vi "synchronize capture with burst.vi"(8 "error in (no error)":errorcluster, 10 "Image Array":T1[](array[typedef]), 11 "Refnum in":T2) -> (0 "error out":errorcluster, 3 "Refnum out":T2)   [LabVIEW 2020]
uses:
  <vilib>/userdefined/High Color/IMAQdx.ctl
  <vilib>/vision/Image Controls.llb/IMAQ Image.ctl
  <vilib>/vision/driver/IMAQdx.llb/IMAQdx Acquisition Mode.ctl
  <vilib>/vision/driver/IMAQdx.llb/IMAQdx Buffer Number Mode.ctl
  <vilib>/vision/driver/NI_Vision_Acquisition_Software.lvlib
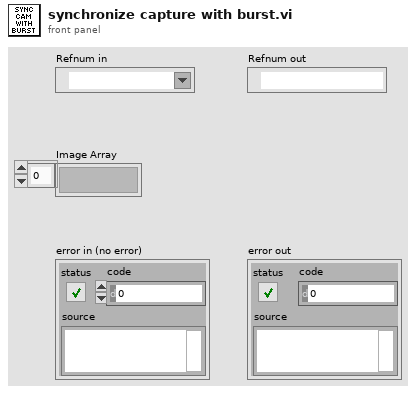
[diagram p1: front panel]
types:
  T1 = typedef "IMAQ Image.ctl" = refnum<image>
  T2 = typedef "IMAQdx.ctl" = refnum<k21>
  T3 = typedef "NI_Vision_Acquisition_Software.lvlib/IMAQdx Acquisition Mode.ctl" = enum32{"One Shot", "Continuous"}
  T4 = typedef "NI_Vision_Acquisition_Software.lvlib/IMAQdx Buffer Number Mode.ctl" = enum32{"Next", "Last", "Buffer Number", "Every", "Last New"}
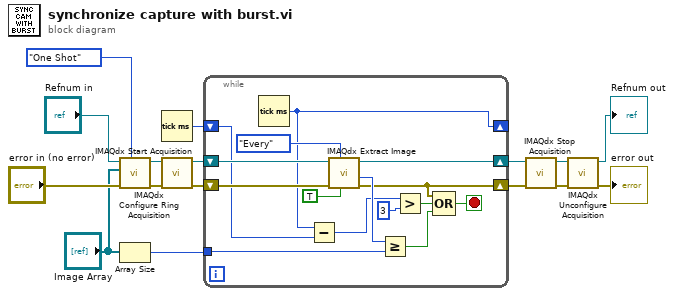
[diagram p0: block diagram]
diagram:
  n1 = call <vilib>:"IMAQdx Configure Ring Acquisition.vi"("Mode"=IMAQdx_Acquisition_Mode."One Shot" ("Continuous?"), "error in"="error in (no error)", "Images"="Image Array", "Session In"="Refnum in") -> ("error out"=w11:errorcluster, "Session Out"=w10:T2)  [unwired: 5 in, 1 out]
  n2 = Array Size(array="Image Array") -> (size(s)=w8:i32)
  n3 = Tick Count (ms)() -> (millisecond timer value=w9:u32)
  n4 = call <vilib>:"IMAQdx Start Acquisition.vi"("error in"=w11, "Session In"=w10) -> ("error out"=w14:errorcluster, "Session Out"=w15:T2)  [unwired: 8 out]
  n5 = while {
    shift-right: [w31] -> w4
    shift-left: w15 -> [w30]
    shift-right: [w17] -> w2
    shift-left: w14 -> [w29]
    shift-right: [w24] -> _
    shift-left: w9 -> [w23]
    tunnel: w8 -> [w25]
    stop <- w18 stop-if-true
    n6 = Tick Count (ms)() -> (millisecond timer value=w24:u32)
    n7 = Subtract(x=w24, y=w23) -> (x-y=w22:u32)
    n8 = call <vilib>:"IMAQdx Extract Image.vi"("Release Previous (true)"=TRUE, "Buffer Number Mode (Next)"=IMAQdx_Buffer_Number_Mode."Every" ("Buffer Number Mode"), "error in"=w29, "Session In"=w30) -> ("error out"=w17:errorcluster, "Buffer Number Out"=w26:u32, "Session Out"=w31:T2)  [unwired: 4 in, 1 out]
    n9 = Greater Or Equal?(x=w26, y=w25) -> (x >= y?=w19:bool)
    n10 = Greater?(x=w22, y=u32 3) -> (0:w20:bool)
    n11 = Compound Arithmetic op=OR(w17, w20, w19) -> (w18:bool)
  }
  n12 = call <vilib>:"IMAQdx Stop Acquisition.vi"("error in"=w2, "Session In"=w4) -> ("error out"=w5:errorcluster, "Session Out"=w6:T2)  [unwired: 8 out]
  n13 = call <vilib>:"IMAQdx Unconfigure Acquisition.vi"("error in"=w5, "Session In"=w6) -> ("error out"=→"error out":errorcluster, "Session Out"=→"Refnum out":T2)  [unwired: 8 out]
